vi "List Mode - Read Configurations for Sequence Setup.vi"   [LabVIEW 2014, in "Associated Power Technologies 8500 Series.lvlib"]
uses:
  <instrlib>/Associated Power Technologies 8500 Series/Associated Power Technologies 8500 Series.lvlib
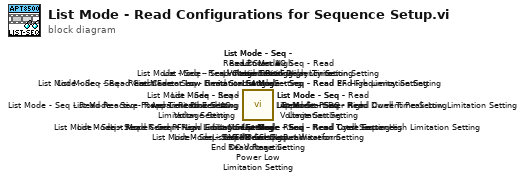
[diagram p0: block diagram]
diagram:
  n1 = call <instrlib>:"List Mode - Seq - Read THD Setting.vi"() -> ()  [unwired: 9 in, 3 out]
  n2 = call <instrlib>:"List Mode - Seq - Read Limitation Delay Time Setting.vi"() -> ()  [unwired: 9 in, 3 out]
  n3 = call <instrlib>:"List Mode - Seq - Read Apparent Power Low Limitation Setting.vi"() -> ()  [unwired: 9 in, 3 out]
  n4 = call <instrlib>:"List Mode - Seq - Read Apparent Power High Limitation Setting.vi"() -> ()  [unwired: 9 in, 3 out]
  n5 = call <instrlib>:"List Mode - Seq - Read Crest Factor Low Limitation Setting.vi"() -> ()  [unwired: 9 in, 3 out]
  n6 = call <instrlib>:"List Mode - Seq - Read Crest Factor High Limitation Setting.vi"() -> ()  [unwired: 9 in, 3 out]
  n7 = call <instrlib>:"List Mode - Seq - Read Reactive Power Low Limitation Setting.vi"() -> ()  [unwired: 9 in, 3 out]
  n8 = call <instrlib>:"List Mode - Seq - Read Reactive Power Limitation Setting.vi"() -> ()  [unwired: 9 in, 3 out]
  n9 = call <instrlib>:"List Mode - Seq - Read Current Peak Low Limitation Setting.vi"() -> ()  [unwired: 9 in, 3 out]
  n10 = call <instrlib>:"List Mode - Seq - Read Current Peak High Limitation Setting.vi"() -> ()  [unwired: 9 in, 3 out]
  n11 = call <instrlib>:"List Mode - Seq - Read PF Low Limitation Setting.vi"() -> ()  [unwired: 9 in, 3 out]
  n12 = call <instrlib>:"List Mode - Seq - Read PF High Limitation Setting.vi"() -> ()  [unwired: 9 in, 3 out]
  n13 = call <instrlib>:"List Mode - Seq - Read Power Low Limitation Setting.vi"() -> ()  [unwired: 9 in, 3 out]
  n14 = call <instrlib>:"List Mode - Seq - Read Power High Limitation Setting.vi"() -> ()  [unwired: 9 in, 3 out]
  n15 = call <instrlib>:"List Mode - Seq - Read Current Low Limitation Setting.vi"() -> ()  [unwired: 9 in, 3 out]
  n16 = call <instrlib>:"List Mode - Seq - Read Current High Limitation Setting.vi"() -> ()  [unwired: 9 in, 3 out]
  n17 = call <instrlib>:"List Mode - Seq - Read Time Unit Setting.vi"() -> ()  [unwired: 9 in, 3 out]
  n18 = call <instrlib>:"List Mode - Seq - Read Dwell Time Setting.vi"() -> ()  [unwired: 9 in, 3 out]
  n19 = call <instrlib>:"List Mode - Seq - Read Cycle Setting.vi"() -> ()  [unwired: 9 in, 3 out]
  n20 = call <instrlib>:"List Mode - Seq - Read End DC Voltage Setting.vi"() -> ()  [unwired: 9 in, 3 out]
  n21 = call <instrlib>:"List Mode - Seq - Read End Frequency Setting.vi"() -> ()  [unwired: 9 in, 3 out]
  n22 = call <instrlib>:"List Mode - Seq - Read End AC Voltage Setting.vi"() -> ()  [unwired: 9 in, 3 out]
  n23 = call <instrlib>:"List Mode - Seq - Read Start DC Voltage Setting.vi"() -> ()  [unwired: 9 in, 3 out]
  n24 = call <instrlib>:"List Mode - Seq - Read Start Frequency Setting.vi"() -> ()  [unwired: 9 in, 3 out]
  n25 = call <instrlib>:"List Mode - Seq - Read Start AC Voltage Setting.vi"() -> ()  [unwired: 9 in, 3 out]
  n26 = call <instrlib>:"List Mode - Seq - Read Start Angle.vi"() -> ()  [unwired: 9 in, 3 out]
  n27 = call <instrlib>:"List Mode - Seq - Read Output Waveform.vi"() -> ()  [unwired: 9 in, 3 out]
  n28 = call <instrlib>:"List Mode - Seq - Read Total Sequences.vi"() -> ()  [unwired: 9 in, 3 out]
  n29 = call <instrlib>:"List Mode - Seq - Read Editing Sequence.vi"() -> ()  [unwired: 9 in, 3 out]
